vi "p8.2.vi"() -> ()   [LabVIEW 2020]
uses:
  <vilib>/vision/NI_Vision_Development_Module.lvlib
panel:
  out "Imagen 1 plano":T1(plugin-control)
  in  "Color Plane":i32(ring)=1 items=["Red", "Green", "Blue", "Hue", "Saturation", "Luminance", "Value", "Intensity"]
  out "Y Resolution":i32=182
  out "X Resolution":i32=202
  out "Histograma Imagen 1 plano":T2(graph)={"Starting Value"=0.0, "Incremental Value"=1.0, "Histogram"=[14531, 4953, 955, 740, 543, 467, 348, 321, 262, 192, 116, 114, 106, 83, 52, 68, 39, 46, 25, 31, 24, 26, 19, 19, 18, 17, 24, 17, 19, 12, 13, 6, 8, 17, 10, 7, 15, 10, 6, 9, 4, 8, 8, 4, 5, 7, 6, 3, 2, 5, 4, 3, 1, 7, 5, 4, 3, 5, 4, 4, 5, 0, 3, 4, 4, 5, 2, 2, 1, 3, 0, 2, 4, 3, 2, 3, 0, 1, 1, 3, 0, 0, 2, 1, 2, 1, 5, 1, 3, 1, 3, 4, 2, 2, 2, 0, 3, 2, 1, 1, 0, 3, 1, 1, 0, 3, 2, 5, 2, 1, 3, 3, 2, 2, 0, 3, 2, 2, 4, 4, 0, 1, 4, 3, 2, 4, 4, 4, 2, 0, 4, 1, 2, 1, 3, 3, 3, 1, 1, 2, 4, 1, 4, 1, 1, 0, 2, 1, 2, 3, 3, 1, 0, 2, 2, 0, 2, 1, 1, 0, 5, 3, 2, 2, 1, 2, 1, 3, 2, 3, 1, 2, 1, 3, 2, 1, 3, 3, 1, 7, 2, 0, 0, 1, 0, 3, 4, 2, 2, 0, 7, 5, 8, 2, 0, 4, 5, 1, 4, 4, 5, 1, 5, 4, 4, 6, 7, 4, 3, 3, 6, 6, 7, 4, 5, 6, 7, 10, 10, 4, 6, 9, 10, 11, 9, 11, 10, 8, 10, 12, 9, 18, 12, 12, 21, 25, 23, 21, 31, 43, 47, 59, 61, 85, 113, 123, 166, 190, 230, 290, 397, 602, 677, 2601, 3647, 2373]}
  out "File Data Type out":i32=8
  out "File Type out":string="JPEG"
  out "error out":errorcluster
  out "Imagen original":T1(plugin-control)
  in  "File Path":path=path "B:/jorge/Desktop/MISC/Curso2021/TDS/laboratorio/P789/imagenes rgb/colores_rgb.jpg"
  in  "Image Type":T3=4 items=["Grayscale (U8)", "Grayscale (I16)", "Grayscale (SGL)", "Complex (CSG)", "RGB (U32)", "HSL (U32)", "RGB (U64)", "Grayscale (U16)"]
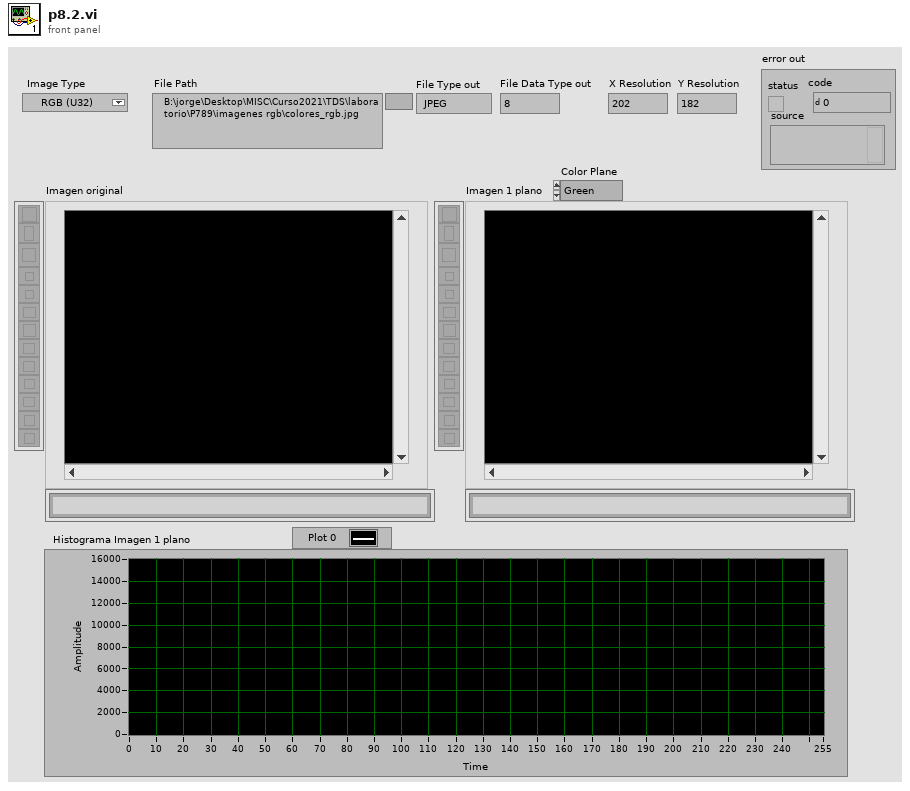
[diagram p1: front panel]
types:
  T1 = typedef "IMAQ Image.ctl" = refnum<image>
  T2 = cluster{"Starting Value":sgl, "Incremental Value":sgl, "Histogram":u32[]}
  T3 = typedef "Image Type" = u32
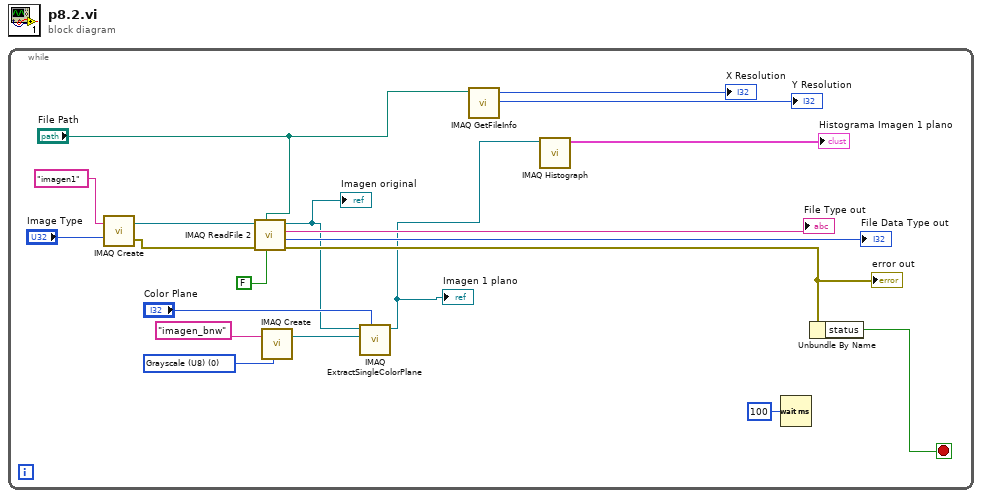
[diagram p0: block diagram]
diagram:
  n1 = while {
    stop <- w15 stop-if-true
    w5 = T3 0 items=["Grayscale (U8)", "Grayscale (I16)", "Grayscale (SGL)", "Complex (CSG)", "RGB (U32)", "HSL (U32)", "RGB (U64)", "Grayscale (U16)"] ("Image Type")
    n2 = call "IMAQ Create"("Image Name"="imagen1", "Image Type"="Image Type") -> ("New Image"=w20:T1, "error out"=w19:errorcluster)  [unwired: 3 in]
    n3 = call "IMAQ ReadFile 2"("Use File Path Image Type"=FALSE, "File Path"="File Path", "error in (no error)"=w19, "Image"=w20) -> ("error out"=w16:errorcluster, "File Data Type out"=→"File Data Type out":i32, "File Type out"=→"File Type out":string, "Image Out"=w1:T1)  [unwired: 3 in, 1 out]
    "Imagen original" <- w1
    "error out" <- w16
    n4 = call "IMAQ Create"("Image Name"="imagen_bnw", "Image Type"=w5) -> ("New Image"=w4:T1)  [unwired: 3 in, 1 out]
    n5 = call "IMAQ ExtractSingleColorPlane"("Color Plane"="Color Plane", "Image Dst"=w4, "Image Src"=w1) -> ("Image Dst Out"=w2:T1)  [unwired: 7 in, 1 out]
    "Imagen 1 plano" <- w2
    n6 = call "IMAQ GetFileInfo"("File Path"="File Path") -> ("Y Resolution"=→"Y Resolution":i32, "X Resolution"=→"X Resolution":i32)  [unwired: 4 in, 5 out]
    n7 = call "IMAQ Histograph"("Image"=w2) -> ("Histogram Graph"=→"Histograma Imagen 1 plano":T2)  [unwired: 7 in, 3 out]
    n8 = Wait (ms)(milliseconds to wait=u32 100) -> ()  [unwired: 1 out]
    n9 = Unbundle By Name(w16) -> ("status"=w15:bool)
  }
